vi "JoinBoolChannel.vi"(11 "Array":bool[](array[boolean])) -> (3 "String":string)   [LabVIEW 2022 SP3]
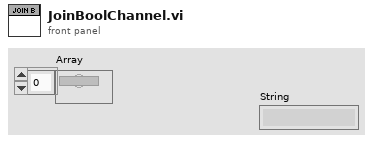
[diagram p1: front panel]
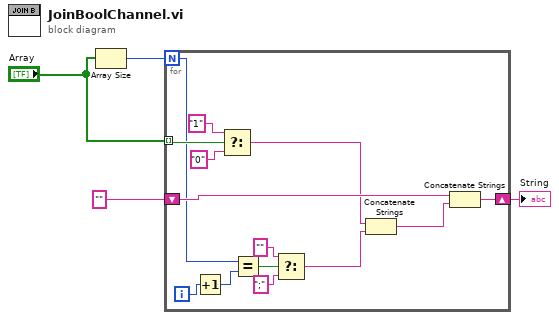
[diagram p0: block diagram]
diagram:
  n1 = Array Size(array="Array") -> (size(s)=w4:i32)
  n2 = for {
    N: w4 -> [w10]
    shift-right: [w18] -> w2
    shift-left: "" -> [w17]
    tunnel: "Array" -> [w16] mode=indexing
    i -> [w12]
    n3 = Increment(x=w12) -> (x+1=w11:i32)
    n4 = Select(t="1", s=w16, f="0") -> (s? t:f=w7:string)
    n5 = Equal?(x=w10, y=w11) -> (x = y?=w13:bool)
    n6 = Select(t="", s=w13, f=";") -> (s? t:f=w6:string)
    n7 = Concatenate Strings(w7, w6) -> (w5:string)
    n8 = Concatenate Strings(w17, w5) -> (w18:string)
  }
  "String" <- w2
